vi "Command_Flywheel.vi"() -> ()   [LabVIEW 2019]
uses:
  Command Execution State.ctl
panel:
  out "Left Speed":dbl
  out "Right Speed":dbl
  out "Completed":bool
  out "Reinit":bool
  in  "Startup":bool
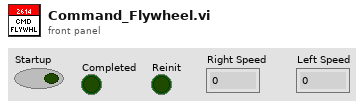
[diagram p1: front panel]
types:
  T1 = typedef "Command Execution State.ctl" = enum16{"Initialize", "Execute", "Finish"}
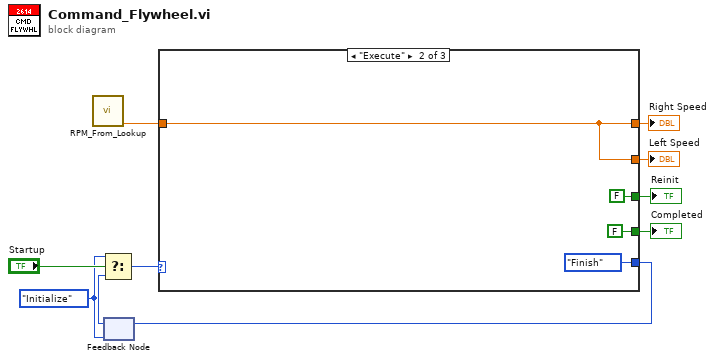
[diagram p0: block diagram]
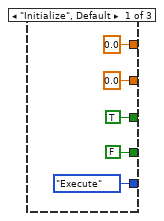
[diagram p2: hidden frame]
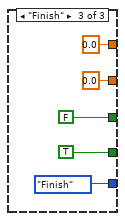
[diagram p3: hidden frame]
diagram:
  w8 = Command_Execution_State."Initialize" ("Play State")
  n1 = call "RPM_From_Lookup.vi"() -> ("RPM output"=w1:dbl)  [unwired: 8 in, 3 out]
  n2 = feedback #1(w8) -> (w7:T1)
  n3 = Select(t=w8, s="Startup", f=w7) -> (s? t:f=w9:T1)
  n4 = case shown="\"Execute\"" w9 {
    tunnel: [TRUE FALSE FALSE] -> w6
    tunnel: [Command_Execution_State."Execute" ("Play State") Command_Execution_State."Finish" ("Play State") Command_Execution_State."Finish" ("Play State")] -> w5
    tunnel: [FALSE FALSE TRUE] -> w4
    tunnel: [0.0 ("Flywheel Speed (RPM)") w16 0.0 ("Flywheel Speed (RPM)")] -> w3
    tunnel: [0.0 ("Flywheel Speed (RPM)") w16 0.0 ("Flywheel Speed (RPM)")] -> w2
    tunnel: w1 -> [_ w16 _]
    frame "Initialize", Default {
    }
    frame "Execute" {
    }
    frame "Finish" {
    }
  }
  "Reinit" <- w6
  "Completed" <- w4
  "Right Speed" <- w2
  "Left Speed" <- w3
  n5 = feedback-in #1(w5) -> ()
